vi "Out_On_N4_X01.vi"(4 "Driver Name":T7, 6 "Error Code":T8, 8 "error in":T6, 11 "DriverConnect in":T1={"InterfaceType"=enum."VISA", "OpenedSession"="", "InterfaceSettings"={"Interface"=enum."RS232", "EOS 4 read"=enum."LF (\\n)", "EOS 4 write"=enum."LF (\\n)", "TMO, ms"=10000, "Sett"=variant(cluster{"Baud Rate":u32, "Data Bits":u16, "Parity":u16, "Stop Bits":u16, "Flow Control":u16, "Eho":bool} {"Baud Rate"=75, "Data Bits"=0, "Parity"=0, "Stop Bits"=0, "Flow Control"=0, "Eho"=FALSE})}}) -> (0 "error out":T6, 3 "DriverConnect out":T1={"InterfaceType"=enum."VISA", "OpenedSession"="", "InterfaceSettings"={"Interface"=enum."RS232", "EOS 4 read"=enum."LF (\\n)", "EOS 4 write"=enum."LF (\\n)", "TMO, ms"=10000, "Sett"=variant(cluster{"Baud Rate":u32, "Data Bits":u16, "Parity":u16, "Stop Bits":u16, "Flow Control":u16, "Eho":bool} {"Baud Rate"=75, "Data Bits"=0, "Parity"=0, "Stop Bits"=0, "Flow Control"=0, "Eho"=FALSE})}})   [LabVIEW 2018]
uses:
  MOKO_LabViewLibrary/MokoLowLevel/MokoLowLovelControl/MLLC_ErrorCode.ctl
  MOKO_LabViewLibrary/MokoLowLevel/MokoLowLovelControl/MLLC_DriverName.ctl
  MOKO_LabViewLibrary/MokoLowLevel/MokoLowLovelControl/MLLC_Error.ctl
  MOKO_LabViewLibrary/MokoLowLevel/MokoLowLovelControl/MLLC_ConnectCluster.ctl
  MOKO_LabViewLibrary/MokoLowLevel/MokoLowLovelControl/MLLC_InterfaceType.ctl
  MOKO_LabViewLibrary/MokoLowLevel/MokoLowLovelControl/MLLC_OpenedSession.ctl
  MOKO_LabViewLibrary/MokoLowLevel/MokoLowLovelControl/MLLC_InterfaceSettings.ctl
  MOKO_LabViewLibrary/MokoLowLevel/MokoLowLovelControl/MLLC_InterfaceKind.ctl
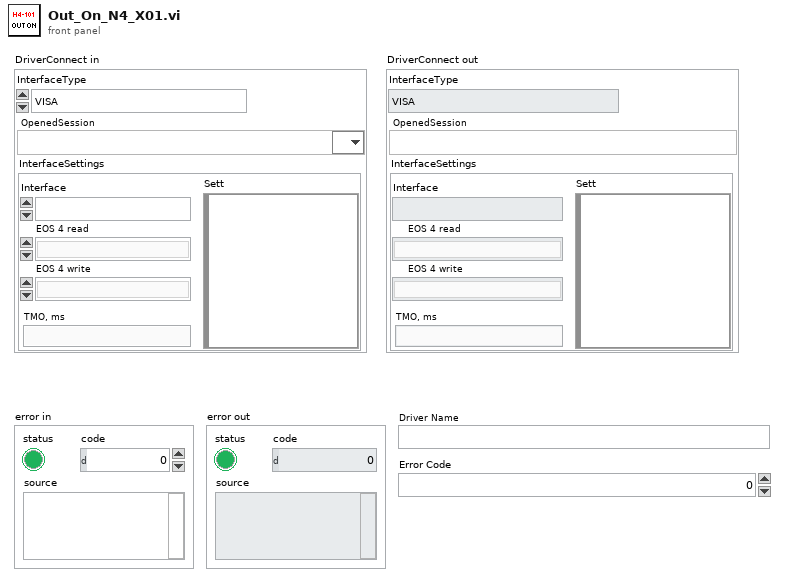
[diagram p1: front panel]
types:
  T1 = typedef "MLLC_ConnectCluster.ctl" = cluster{"InterfaceType":T2, "OpenedSession":T3, "InterfaceSettings":T4}
  T2 = typedef "MLLC_InterfaceType.ctl" = enum16{"VISA", "Prologix USB-GPIB"}
  T3 = typedef "MLLC_OpenedSession.ctl" = refnum<visa-resource-name>
  T4 = typedef "MLLC_InterfaceSettings.ctl" = cluster{"Interface":T5, "EOS 4 read":enum16{"Default (=EOS 4 write)", "CR (\\r)", "LF (\\n)", "None"}, "EOS 4 write":enum16{"CR+LF (\\r\\n)", "CR (\\r)", "LF (\\n)", "None"}, "TMO, ms":i32, "Sett":variant}
  T5 = typedef "MLLC_InterfaceKind.ctl" = enum16{"RS232", "GPIB", "USB", "Ethernet", "another"}
  T6 = typedef "MLLC_Error.ctl" = errorcluster
  T7 = typedef "MLLC_DriverName.ctl" = string
  T8 = typedef "MLLC_ErrorCode.ctl" = u32
  T9 = typedef "MLLC_Response.ctl" = string
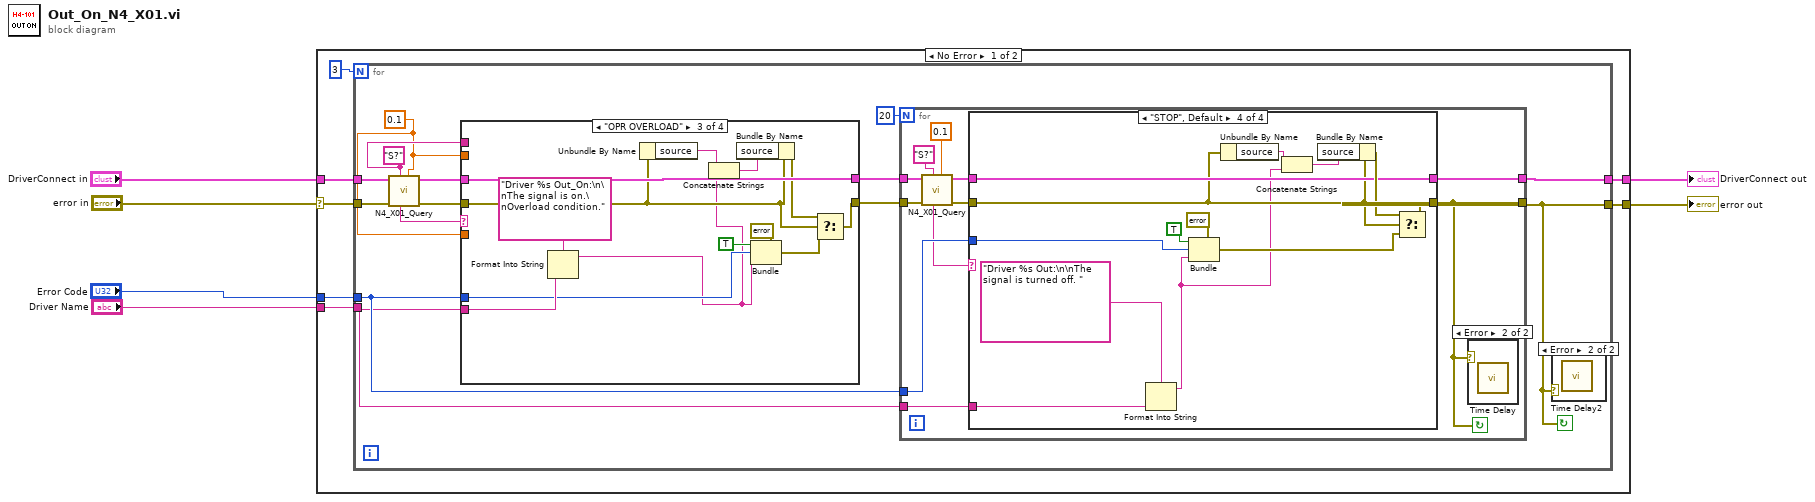
[diagram p0: block diagram]
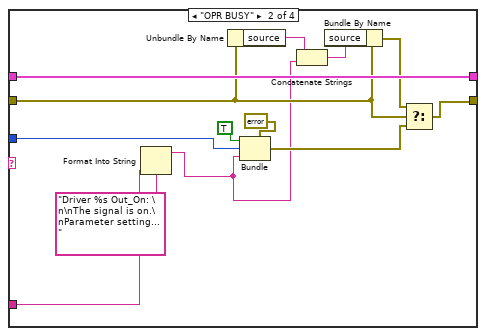
[diagram p3: hidden frame]
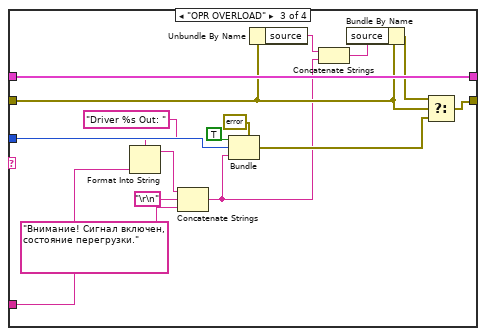
[diagram p4: hidden frame]
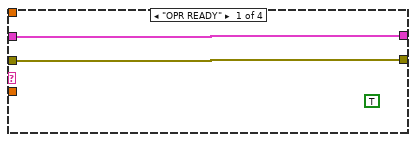
[diagram p7: hidden frame]
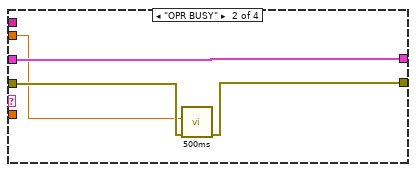
[diagram p8: hidden frame]
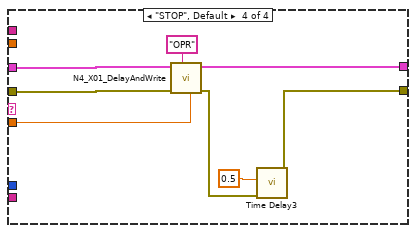
[diagram p9: hidden frame]
diagram:
  n1 = case shown="No Error" "error in" {
    selector: "error in" -> [w7 w110]
    tunnel: "DriverConnect in" -> [w8 w111]
    tunnel: [w11 w111] -> w1
    tunnel: [w10 w110] -> w3
    tunnel: "Driver Name" -> [w12 _]
    tunnel: "Error Code" -> [w13 _]
    frame No Error {
      n2 = for {
        N: 3 -> [_]
        tunnel: w13 -> [w22]
        tunnel: w12 -> [w21]
        tunnel: [w20] -> w11
        tunnel: [w17] -> w10
        tunnel: w8 -> [w19]
        tunnel: w7 -> [w18]
        stop <- w17 continue-if-true
        w15 = 0.1 ("Delay Time (s)")
        w16 = "S?" ("Error Query")
        n3 = call "N4_X01_Query.vi"("Delay Befor (s)"=w15, "Command"=w16, "error in"=w18, "DriverConnect in"=w19) -> ("error out"=w25:T6, "DriverConnect out"=w26:T1, "Response"=w27:T9)  [unwired: 5 in]
        n4 = case shown="\"OPR OVERLOAD\"" w27 {
          tunnel: w26 -> [w84 w88 w98 w108]
          tunnel: w25 -> [w83 w86 w92 w107]
          tunnel: [w84 w88 w98 w103] -> w24
          tunnel: [w83 w87 w90 w104] -> w23
          tunnel: w21 -> [_ _ w101 _]
          tunnel: w22 -> [_ _ w100 _]
          tunnel: w15 -> [_ _ _ w106]
          tunnel: w16 -> [_ _ _ _]
          tunnel: w15 -> [_ w85 _ _]
          frame "OPR READY" {
            (unwired) TRUE
          }
          frame "OPR BUSY" {
            n5 = call "500ms"("error in (no error)"=w86, "Delay Time (s)"=w85) -> ("error out"=w87:errorcluster)  [unwired: 9 in]
          }
          frame "OPR OVERLOAD" {
            n6 = Format Into String(format string="Driver %s Out_On:\n\nThe signal is on.\nOverload condition.", w101) -> (resulting string=w89:string)  [unwired: 2 in, 1 out]
            n7 = Unbundle By Name(w92) -> ("source"=w96:string)
            n8 = Concatenate Strings(w96, w89) -> (w95:string)
            n9 = Bundle By Name(cluster=w92, "source"=w95) -> (w91:T6)
            n10 = Bundle(cluster=errorcluster {"status"=FALSE, "code"=0, "source"=""} ("error out"), "status"=TRUE ("Status"), "code"=w100, "source"=w89) -> (w93:errorcluster)
            n11 = Select(t=w91, s=w92, f=w93) -> (s? t:f=w90:T6)
          }
          frame "STOP", Default {
            n12 = call "N4_X01_DelayAndWrite.vi"("Delay Befor (s)"=w106, "Command"="OPR" ("String"), "error in"=w107, "DriverConnect in"=w108) -> ("error out"=w105:T6, "DriverConnect out"=w103:T1)  [unwired: 6 in]
            n13 = call "Time Delay3"("error in (no error)"=w105, "Delay Time (s)"=0.5) -> ("error out"=w104:errorcluster)  [unwired: 9 in]
          }
        }
        n14 = for {
          N: 20 -> [_]
          tunnel: w24 -> [w36]
          tunnel: w23 -> [w35]
          tunnel: [w32] -> w20
          tunnel: [w31] -> w17
          tunnel: w22 -> [w30]
          tunnel: w21 -> [w29]
          stop <- w31 continue-if-true
          n15 = call "N4_X01_Query.vi"("Delay Befor (s)"=0.1 ("Delay Time (s)"), "Command"="S?" ("Error Query"), "error in"=w35, "DriverConnect in"=w36) -> ("error out"=w33:T6, "DriverConnect out"=w34:T1, "Response"=w28:T9)  [unwired: 5 in]
          n16 = case shown="\"STOP\", Default" w28 {
            tunnel: w34 -> [w40 w53 w62 w72]
            tunnel: w33 -> [w39 w45 w55 w71]
            tunnel: [w40 w53 w62 w72] -> w32
            tunnel: [w39 w42 w58 w74] -> w31
            tunnel: w29 -> [_ w50 w65 w81]
            tunnel: w30 -> [_ w51 w64 w80]
            frame "OPR READY" {
            }
            frame "OPR BUSY" {
              n17 = Format Into String(format string="Driver %s Out_On: \n\nThe signal is on.\nParameter setting...", w50) -> (resulting string=w41:string)  [unwired: 2 in, 1 out]
              n18 = Unbundle By Name(w45) -> ("source"=w48:string)
              n19 = Bundle(cluster=errorcluster {"status"=FALSE, "code"=0, "source"=""} ("error out"), "status"=TRUE ("Status"), "code"=w51, "source"=w41) -> (w43:errorcluster)
              n20 = Concatenate Strings(w48, w41) -> (w47:string)
              n21 = Bundle By Name(cluster=w45, "source"=w47) -> (w46:T6)
              n22 = Select(t=w46, s=w45, f=w43) -> (s? t:f=w42:T6)
            }
            frame "OPR OVERLOAD" {
              n23 = Format Into String(format string="Driver %s Out: ", w65) -> (resulting string=w67:string)  [unwired: 2 in, 1 out]
              n24 = Concatenate Strings(w67, "\r\n", "Внимание! Сигнал включен, состояние перегрузки." ("string")) -> (w54:string)
              n25 = Bundle(cluster=errorcluster {"status"=FALSE, "code"=0, "source"=""} ("error out"), "status"=TRUE ("Status"), "code"=w64, "source"=w54) -> (w59:errorcluster)
              n26 = Unbundle By Name(w55) -> ("source"=w56:string)
              n27 = Concatenate Strings(w56, w54) -> (w61:string)
              n28 = Bundle By Name(cluster=w55, "source"=w61) -> (w57:T6)
              n29 = Select(t=w57, s=w55, f=w59) -> (s? t:f=w58:T6)
            }
            frame "STOP", Default {
              n30 = Format Into String(format string="Driver %s Out:\n\nThe signal is turned off. ", w81) -> (resulting string=w70:string)  [unwired: 2 in, 1 out]
              n31 = Bundle(cluster=errorcluster {"status"=FALSE, "code"=0, "source"=""} ("error out"), "status"=TRUE ("Status"), "code"=w80, "source"=w70) -> (w75:errorcluster)
              n32 = Unbundle By Name(w71) -> ("source"=w76:string)
              n33 = Concatenate Strings(w76, w70) -> (w78:string)
              n34 = Bundle By Name(cluster=w71, "source"=w78) -> (w77:T6)
              n35 = Select(t=w77, s=w71, f=w75) -> (s? t:f=w74:T6)
            }
          }
          n36 = case shown="Error" w31 {
            frame No Error {
            }
            frame Error {
              n37 = call "Time Delay"() -> ()  [unwired: 11 in, 1 out]
            }
          }
        }
        n38 = case shown="Error" w17 {
          frame No Error {
          }
          frame Error {
            n39 = call "Time Delay2"() -> ()  [unwired: 11 in, 1 out]
          }
        }
      }
    }
    frame Error {
    }
  }
  "error out" <- w3
  "DriverConnect out" <- w1
